vi "Acquisition_b.vi"() -> (4 "Acquired_Data":dbl(graph))   [LabVIEW 2023]
doc: "This VI acquire data that were generated be the Generator VI.\nTransfer of thet data happens under Simple LV2."
uses:
  Controls/Operation_Simple_LV2.ctl
panel:
  out "Error_Out":errorcluster
  in  "Error_In":errorcluster
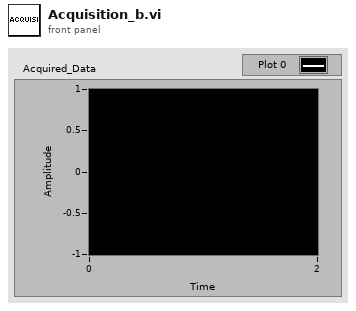
[diagram p1: front panel]
types:
  T1 = typedef "Operation_Simple_LV2.ctl" = enum16{"Write", "Read"}
  T2 = enum16{"Left Button", "Center Button", "Right Button", "Window Close"}
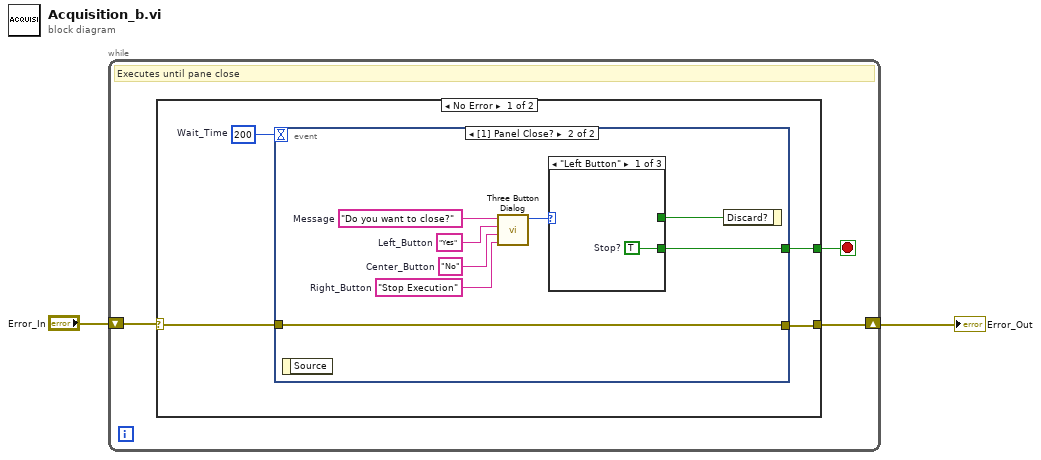
[diagram p0: block diagram]
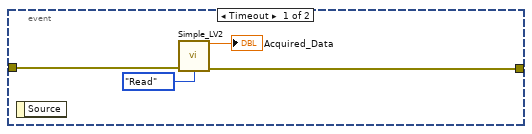
[diagram p2: hidden frame]
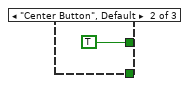
[diagram p3: hidden frame]
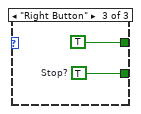
[diagram p4: hidden frame]
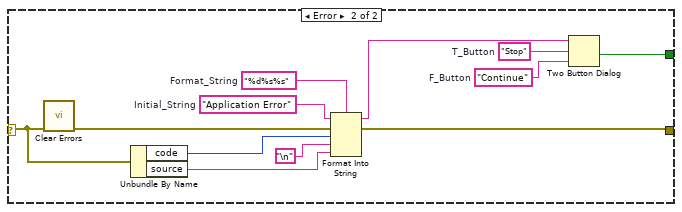
[diagram p5: hidden frame]
diagram:
  n1 = while {
    shift-right: [w3] -> w1
    shift-left: "Error_In" -> [w4]
    stop <- w5 stop-if-true
    # "Executes until pane close"
    n2 = case shown="No Error" w4 {
      selector: w4 -> [w7 w30]
      tunnel: [w8 w26] -> w5
      tunnel: [w6 w31] -> w3
      frame No Error {
        w9 = 200  # Wait_Time
        n3 = event shown="[1] Panel Close?" {
          selector: _ -> [_ _]
          dyn-events: _ -> [_ _]
          timeout: w9 -> [_ _]
          tunnel: [_ w15] -> w8
          tunnel: w7 -> [w12 w14]
          tunnel: [w11 w14] -> w6
          event Timeout {
            n4 = event-data() -> ()  [unwired: 1 in, 1 out]
            n5 = call "Simple_LV2.vi"("Error_In"=w12, "Operation"=Operation_Simple_LV2."Read") -> ("Data_Out"=→"Acquired_Data":dbl, "Error_Out"=w11:errorcluster)  [unwired: 12 in]
          }
          event Panel Close? {
            w18 = "Stop Execution"  # Right_Button
            w19 = "No"  # Center_Button
            w20 = "Yes"  # Left_Button
            w21 = "Do you want to close?"  # Message
            n6 = event-data() -> ()  [unwired: 1 in, 1 out]
            n7 = call <vilib>:"Three Button Dialog.vi"("Right Button Text (\"Cancel\")"=w18, "Center Button Text (\"No\")"=w19, "Left Button Text (\"Yes\")"=w20, "message"=w21) -> ("Which Button?"=w17:T2)  [unwired: 7 in]
            n8 = case shown="\"Left Button\"" w17 {
              tunnel: [_ TRUE ("Discard?") TRUE ("Discard?")] -> w16
              tunnel: [w22 _ w25] -> w15
              frame "Left Button" {
                w22 = TRUE  # Stop?
              }
              frame "Center Button", Default {
              }
              frame "Right Button" {
                w25 = TRUE  # Stop?
              }
            }
            n9 = event-data("Discard?"=w16) -> ()  [unwired: 1 in, 1 out]
          }
        }
      }
      frame Error {
        w33 = "%d%s%s"  # Format_String
        w34 = "Application Error"  # Initial_String
        w35 = "Stop"  # T_Button
        w36 = "Continue"  # F_Button
        n10 = call <vilib>:"Clear Errors.vi"("error in (no error)"=w30) -> ("error out"=w29:errorcluster)  [unwired: 5 in, 1 out]
        n11 = Unbundle By Name(w30) -> ("code"=w28:i32, "source"=w27:string)
        n12 = Format Into String(format string=w33, initial string=w34, error in=w29, w28, "\n", w27) -> (resulting string=w37:string, error out=w31:errorcluster)
        n13 = Two Button Dialog(message=w37, 1:w36, 2:w35) -> (T button?=w26:bool)
      }
    }
  }
  "Error_Out" <- w1
